vi "WFDC Setup Camera.vi"(0 "Base Data Path":path=path "C:/Users/George Sirinakis/Documents/Microscope Control/Microscope Modules/Wide Field Drift Correction/WFDC Default Data Storage", 7 "Camera Notifier Name":string, 13 "ROI File Name":string="ROI File Name") -> (4 "Current Save Path":path, 8 "Canceled?":bool)   [LabVIEW 2016]
uses:
  Device Library/Cameras/IDS/IDS Controls/IDS Actions.ctl
  Device Library/Cameras/IDS/IDS Controls/IDS Parameters.ctl
  Device Library/Cameras/IDS/IDS Controls/IDS Parameter List.ctl
  Device Library/Cameras/IDS/IDS Controls/IDS ROI.ctl
  <vilib>/Utility/miscctls.llb/LVPointTypeDef.ctl
panel:
  in  "Exposure Time (ms)":dbl
  in  "Tool Selection":enum32{"Zoom Tool", "ROI Tool", "Pan Tool"}(radio)
  in  "Cancel":bool
  in  "Done":bool
  out "Camera Display":T1(plugin-control)
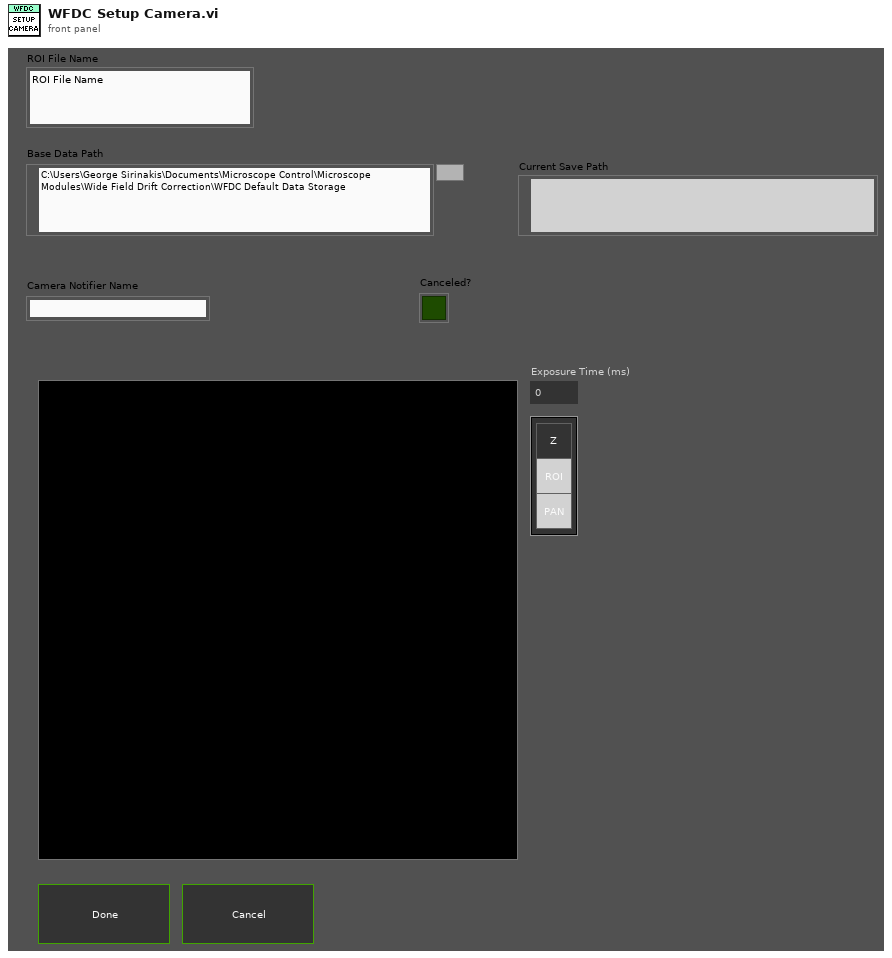
[diagram p1: front panel]
types:
  T1 = typedef "IMAQ Image.ctl" = refnum<image>
  T2 = enum16{"Always On", "Always Off", "Off While Running"}
  T3 = typedef "LVPointTypeDef.ctl" = cluster{"Horizontal":i16, "Vertical":i16}
  T4 = typedef "IDS ROI.ctl" = cluster{"H Offset":i32, "V Offset":i32, "H Width":i32, "V Width":i32}
  T5 = typedef "IDS Actions.ctl" = enum16{"Error Check", "Initialize", "Preview", "Record", "Abort", "Record Settings", "Set Parameter", "Get Parameter", "Set ROI", "Get ROI", "Status", "Quit"}
  T6 = typedef "IDS Parameters.ctl" = cluster{"Parameter":T7, "Value":dbl}
  T7 = typedef "IDS Parameter List.ctl" = enum16{"Exposure Time (s)"}
  T8 = typedef "LVRectTypeDef.ctl" = cluster{"Left":i16, "Top":i16, "Right":i16, "Bottom":i16}
  T9 = typedef "LVBoundsTypeDef.ctl" = cluster{"Width":u32, "Height":u32}
  T10 = cluster{"Global Rectangle":i32[], "Contours":cluster{"Contour Type":u32, "ROI Type":u32, "Points":i32[]}[]}
  T11 = cluster{"Contour Type":u32, "ROI Type":u32, "Points":i32[]}[]
  T12 = cluster{"Contour Type":u32, "ROI Type":u32, "Points":i32[]}
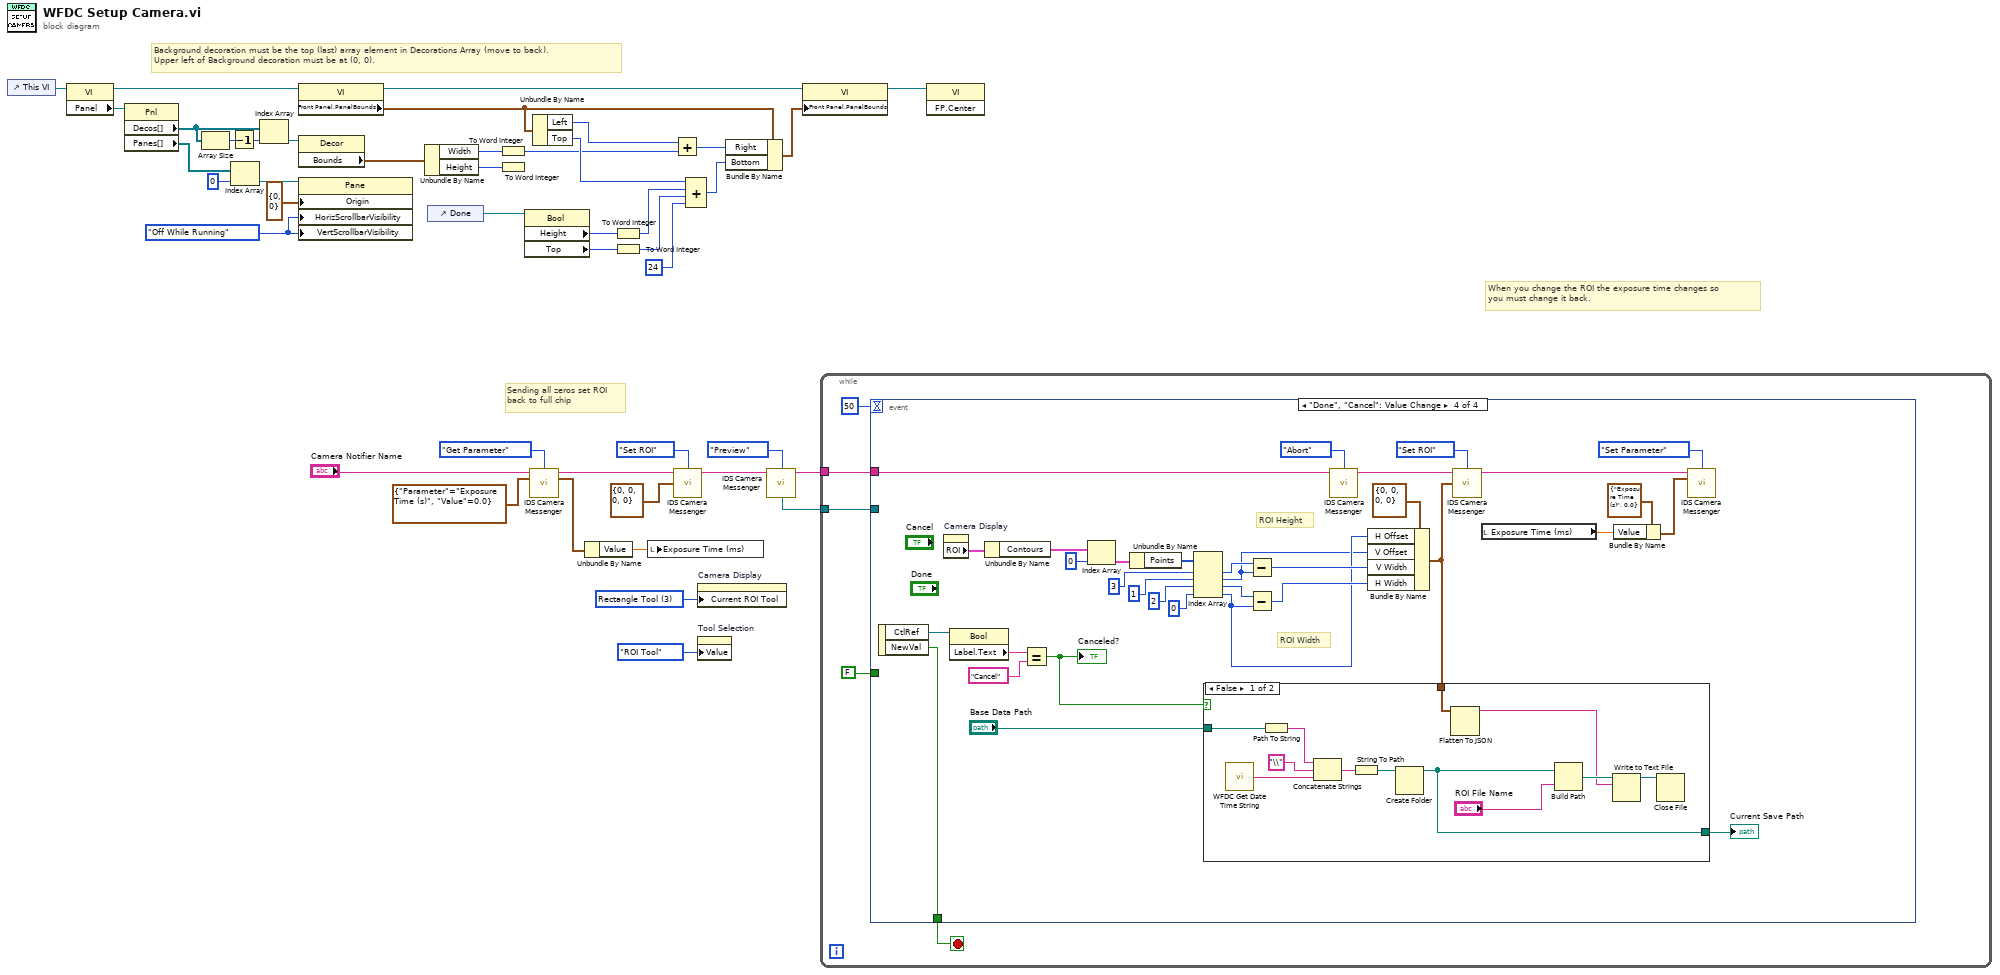
[diagram p0: block diagram]
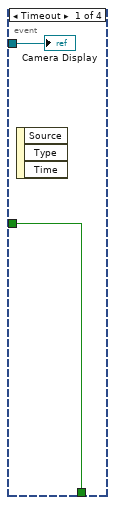
[diagram p2: hidden frame]
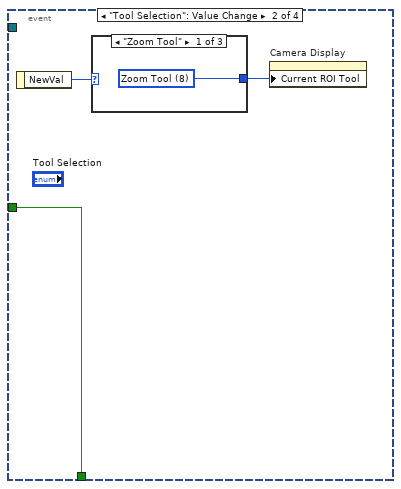
[diagram p3: hidden frame]
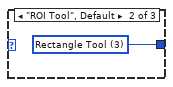
[diagram p4: hidden frame]
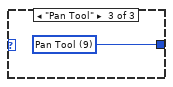
[diagram p5: hidden frame]
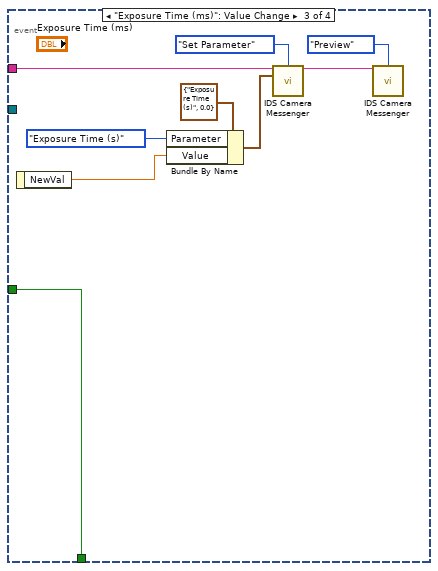
[diagram p6: hidden frame]
diagram:
  w13 = T2."Off While Running" ("Vertical Scrollbar Visibility")
  w36 = u32 3 items=["Zoom Tool"=8, "Selection Tool"=0, "Pan Tool"=9, "Point Tool"=1, "Line Tool"=2, "Rectangle Tool"=3, "Rotated Rectangle Tool"=12, "Polyline Tool"=10, "Polygon Tool"=5, "Freehand Tool"=11, "Closed Freehand Tool"=6, "Ellipse Tool"=4, "Annulus Tool"=7] ("Current ROI Tool")
  # "Background decoration must be the top (last) array element in Decorations Array (move to back).\nUpper left of Background decoration must be at (0, 0)."
  # "When you change the ROI the exposure time changes so\nyou must change it back."
  # "Sending all zeros set ROI\nback to full chip"
  n1 = control-ref of="This VI"() -> (w5:refnum<vi>)
  n2 = property class="VI"(reference=w5) -> (reference out=w14:refnum<vi>, "Panel"=w6:refnum<vi>)  [unwired: 1 in, 1 out]
  n3 = property class="Pnl"(reference=w6) -> ("Decos[]"=w4:refnum<vi>[], "Panes[]"=w10:refnum<vi>[])  [unwired: 1 in, 2 out]
  n4 = Array Size(array=w4) -> (size(s)=w2:i32)
  n5 = Decrement(x=w2) -> (x-1=w3:i32)
  n6 = Index Array(array=w10, index=0) -> (element=w9:refnum<vi>)
  n7 = Index Array(array=w4, index=w3) -> (element=w12:refnum<vi>)
  n8 = property class="VI"(reference=w14) -> (reference out=w16:refnum<vi>, "Front Panel.PanelBounds"=w17:T8)  [unwired: 1 in, 1 out]
  n9 = property class="Decor"(reference=w12) -> ("Bounds"=w15:T9)  [unwired: 1 in, 2 out]
  n10 = property class="Pane"(reference=w9, "Origin"=T3 {"Horizontal"=0, "Vertical"=0}, "HorizScrollbarVisibility"=w13, "VertScrollbarVisibility"=w13) -> ()  [unwired: 1 in, 2 out]
  n11 = Unbundle By Name(w15) -> ("Width"=w20:u32, "Height"=w23:u32)
  n12 = control-ref of="Done"() -> (w7:refnum<vi>)
  n13 = To Word Integer(number=w20) -> (16bit integer=w22:i16)
  n14 = To Word Integer(number=w23) -> ()  [unwired: 1 out]
  n15 = property class="Bool"(reference=w7) -> ("Height"=w25:u32, "Top"=w26:i32)  [unwired: 1 in, 2 out]
  n16 = call "IDS Camera Messenger.vi"("Notifier Name"="Camera Notifier Name", "IDS Actions"=IDS_Actions."Get Parameter", "IDS Parameter"=T6 {"Parameter"=enum."Exposure Time (s)", "Value"=0.0}) -> ("Notifier Name (Dup)"=w33:string, "IDS Parameter"=w38:T6)  [unwired: 7 in, 4 out]
  n17 = Unbundle By Name(w17) -> ("Left"=w19:i16, "Top"=w30:i16)
  n18 = Unbundle By Name(w38) -> ("Value"=w37:dbl)
  n19 = To Word Integer(number=w25) -> (16bit integer=w28:i16)
  n20 = To Word Integer(number=w26) -> (16bit integer=w29:i16)
  n21 = local write "Exposure Time (ms)"(w37) -> ()
  n22 = Add(x=w19, y=w22) -> (x+y=w21:i16)
  n23 = call "IDS Camera Messenger.vi"("Notifier Name"=w33, "IDS Actions"=IDS_Actions."Set ROI", "ROI Setup"=T4 {"H Offset"=0, "V Offset"=0, "H Width"=0, "V Width"=0}) -> ("Notifier Name (Dup)"=w32:string)  [unwired: 7 in, 5 out]
  n24 = Compound Arithmetic op=ADD(w30, w28, w29, i16 24 ("y")) -> (w24:i16)
  n25 = property on="Camera Display" class="ImageControl"("Current ROI Tool"=w36) -> ()  [unwired: 2 in, 2 out]
  n26 = property on="Tool Selection" class="RadioBtnsControl (strict)"("Value"=enum32{"Zoom Tool", "ROI Tool", "Pan Tool"}."ROI Tool" ("Tool Selection")) -> ()  [unwired: 2 in, 2 out]
  n27 = Bundle By Name(cluster=w17, "Right"=w21, "Bottom"=w24) -> (w18:T8)
  n28 = call "IDS Camera Messenger.vi"("Notifier Name"=w32, "IDS Actions"=IDS_Actions."Preview") -> ("Notifier Name (Dup)"=w42:string, "Image Ref"=w43:T1)  [unwired: 8 in, 4 out]
  n29 = property class="VI"(reference=w16, "Front Panel.PanelBounds"=w18) -> (reference out=w1:refnum<vi>)  [unwired: 1 in, 1 out]
  n30 = while {
    tunnel: w43 -> [w47]
    tunnel: w42 -> [w45]
    stop <- w49 stop-if-true
    n31 = event shown="[3] \"Done\", \"Cancel\": Value Change" {
      selector: _ -> [_ _ _ _]
      dyn-events: _ -> [_ _ _ _]
      timeout: 50 -> [_ _ _ _]
      tunnel: [w51 w54 w66 w96] -> w49
      tunnel: FALSE -> [w51 w54 w66 _]
      tunnel: w47 -> [w50 _ _ _]
      tunnel: w45 -> [_ _ w64 w94]
      event Timeout {
        n32 = event-data() -> ()  [unwired: 1 in, 3 out]
        "Camera Display" <- w50
      }
      event "Tool Selection": Value Change {
        n33 = event-data() -> ("NewVal"=w53:enum32{"Zoom Tool", "ROI Tool", "Pan Tool"})  [unwired: 1 in]
        n34 = case shown="\"Zoom Tool\"" w53 {
          tunnel: [w55 w56 w57] -> w52
          frame "Zoom Tool" {
            w55 = u32 8 items=["Zoom Tool"=8, "Selection Tool"=0, "Pan Tool"=9, "Point Tool"=1, "Line Tool"=2, "Rectangle Tool"=3, "Rotated Rectangle Tool"=12, "Polyline Tool"=10, "Polygon Tool"=5, "Freehand Tool"=11, "Closed Freehand Tool"=6, "Ellipse Tool"=4, "Annulus Tool"=7] ("Current ROI Tool")
          }
          frame "ROI Tool", Default {
            w56 = u32 3 items=["Zoom Tool"=8, "Selection Tool"=0, "Pan Tool"=9, "Point Tool"=1, "Line Tool"=2, "Rectangle Tool"=3, "Rotated Rectangle Tool"=12, "Polyline Tool"=10, "Polygon Tool"=5, "Freehand Tool"=11, "Closed Freehand Tool"=6, "Ellipse Tool"=4, "Annulus Tool"=7] ("Current ROI Tool")
          }
          frame "Pan Tool" {
            w57 = u32 9 items=["Zoom Tool"=8, "Selection Tool"=0, "Pan Tool"=9, "Point Tool"=1, "Line Tool"=2, "Rectangle Tool"=3, "Rotated Rectangle Tool"=12, "Polyline Tool"=10, "Polygon Tool"=5, "Freehand Tool"=11, "Closed Freehand Tool"=6, "Ellipse Tool"=4, "Annulus Tool"=7] ("Current ROI Tool")
          }
        }
        n35 = property on="Camera Display" class="ImageControl"("Current ROI Tool"=w52) -> ()  [unwired: 2 in, 2 out]
      }
      event "Exposure Time (ms)": Value Change {
        n36 = event-data() -> ("NewVal"=w60:dbl)  [unwired: 1 in]
        n37 = Bundle By Name(cluster=T6 {"Parameter"=enum."Exposure Time (s)", "Value"=0.0} ("IDS Parameter"), "Parameter"=IDS_Parameter_List."Exposure Time (s)", "Value"=w60) -> (w61:T6)
        n38 = call "IDS Camera Messenger.vi"("Notifier Name"=w64, "IDS Actions"=IDS_Actions."Set Parameter", "IDS Parameter"=w61) -> ("Notifier Name (Dup)"=w58:string)  [unwired: 7 in, 5 out]
        n39 = call "IDS Camera Messenger.vi"("Notifier Name"=w58, "IDS Actions"=IDS_Actions."Preview") -> ()  [unwired: 8 in, 6 out]
      }
      event "Done", "Cancel": Value Change {
        # "ROI Width"
        # "ROI Height"
        n40 = event-data() -> ("CtlRef"=w99:refnum<vi>, "NewVal"=w96:bool)  [unwired: 1 in]
        n41 = property on="Camera Display" class="ImageControl"() -> ("ROI"=w90:T10)  [unwired: 2 in, 2 out]
        n42 = property class="Bool"(reference=w99) -> ("Label.Text"=w98:string)  [unwired: 1 in, 2 out]
        n43 = Unbundle By Name(w90) -> ("Contours"=w89:T11)
        n44 = Equal?(x=w98, y="Cancel") -> (x = y?=w70:bool)
        "Canceled?" <- w70
        n45 = Index Array(array=w89, index=0) -> (element=w88:T12)
        n46 = Unbundle By Name(w88) -> ("Points"=w91:i32[])
        n47 = Index Array(array=w91, index #1=3 ("index"), index #2=1 ("index"), index #3=2 ("index"), index #4=0 ("index")) -> (element #1=w93:i32, element #2=w84:i32, element #3=w92:i32, element #4=w85:i32)
        n48 = Subtract(x=w93, y=w84) -> (x-y=w87:i32)
        n49 = Subtract(x=w92, y=w85) -> (x-y=w86:i32)
        n50 = call "IDS Camera Messenger.vi"("Notifier Name"=w94, "IDS Actions"=IDS_Actions."Abort") -> ("Notifier Name (Dup)"=w76:string)  [unwired: 8 in, 5 out]
        n51 = Bundle By Name(cluster=T4 {"H Offset"=0, "V Offset"=0, "H Width"=0, "V Width"=0} ("ROI Setup"), "H Offset"=w85, "V Offset"=w84, "V Width"=w87, "H Width"=w86) -> (w69:T4)
        n52 = case shown="False" w70 {
          tunnel: w69 -> [w105 _]
          tunnel: "Base Data Path" -> [w102 w112]
          tunnel: [w101 w112] -> w67
          frame False {
            n53 = call "WFDC Get Date Time String.vi"() -> ("Date Time String"=w100:string)  [unwired: 15 in]
            n54 = Path To String(path=w102) -> (string=w109:string)
            n55 = Concatenate Strings(w109, "\\" ("regular expression"), w100) -> (w110:string)
            n56 = String To Path(string=w110) -> (path=w111:path)
            n57 = Create Folder(path (use dialog)=w111) -> (created path=w101:path)  [unwired: 2 in, 2 out]
            n58 = Flatten To JSON(anything=w105) -> (JSON string=w104:string)  [unwired: 2 in, 1 out]
            n59 = Build Path(base path=w101, name or relative path="ROI File Name") -> (appended path=w106:path)
            n60 = Write to Text File(file (use dialog)=w106, text=w104) -> (refnum out=w107:refnum<file>)  [unwired: 2 in, 2 out]
            n61 = Close File(refnum=w107) -> ()  [unwired: 1 in, 2 out]
          }
          frame True {
          }
        }
        "Current Save Path" <- w67
        n62 = call "IDS Camera Messenger.vi"("Notifier Name"=w76, "IDS Actions"=IDS_Actions."Set ROI", "ROI Setup"=w69) -> ("Notifier Name (Dup)"=w74:string)  [unwired: 7 in, 5 out]
        n63 = local read "Exposure Time (ms)"() -> (w73:dbl)
        n64 = Bundle By Name(cluster=T6 {"Parameter"=enum."Exposure Time (s)", "Value"=0.0} ("IDS Parameter"), "Value"=w73) -> (w71:T6)
        n65 = call "IDS Camera Messenger.vi"("Notifier Name"=w74, "IDS Actions"=IDS_Actions."Set Parameter", "IDS Parameter"=w71) -> ()  [unwired: 7 in, 6 out]
      }
    }
  }
  n66 = invoke class="VI" method="FP.Center"(reference=w1) -> ()  [unwired: 2 in, 3 out]
